vi "430_TCP_compound query test.vi"() -> ()   [LabVIEW 2011]
panel:
  out "refnum out":refnum<file>
  out "file check":errorcluster
  in  "file path (use dialog)":path
  in  "save":bool
  out "status":i32
  in  "Timeout":i32=1000
  out "field":string
  out "Query check":errorcluster
  out "Response":string
  in  "Command":string
  out "Init Response":string
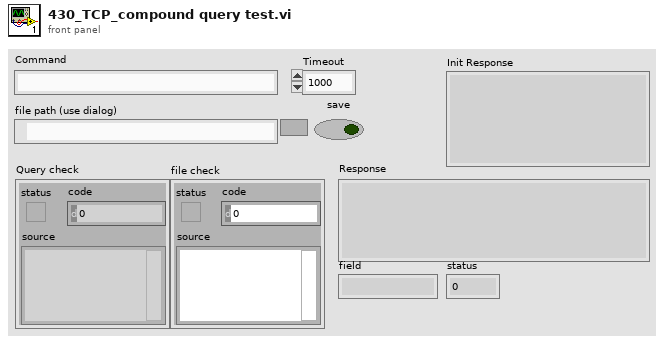
[diagram p1: front panel]
types:
  T1 = enum16{"open", "replace", "create", "open or create", "replace or create", "replace or create with confirmation"}
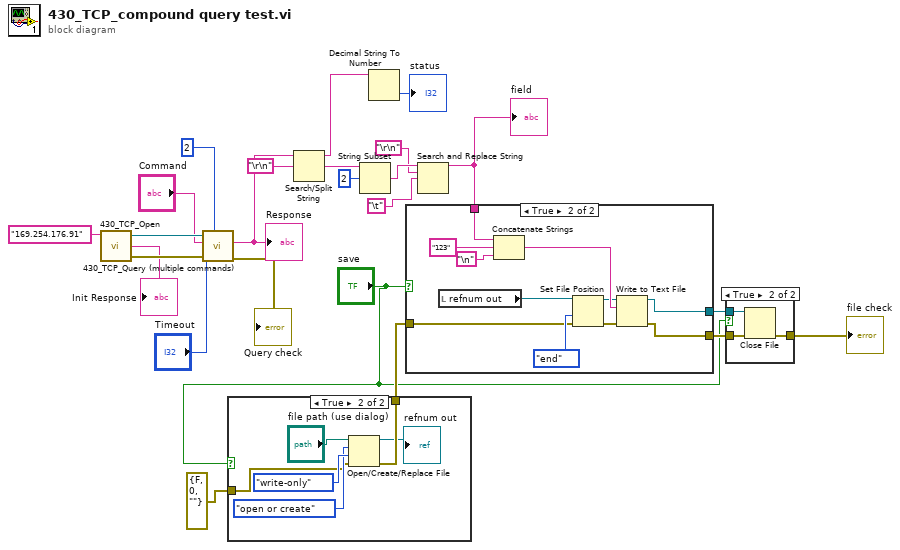
[diagram p0: block diagram]
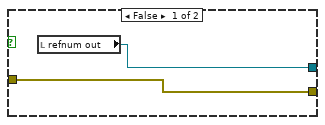
[diagram p4: hidden frame]
diagram:
  n1 = call "430_TCP_Open.vi"("IP Address"="169.254.176.91") -> ("connection ID"=w22:refnum<k5>, "Init Response"=→"Init Response":string, "error out"=w23:errorcluster)  [unwired: 5 in]
  n2 = call "430_TCP_Query (multiple commands).vi"("Number of\nquerys"=2 ("Number of\nquerys"), "error in (no error)"=w23, "Timeout"="Timeout", "Command"="Command", "connection ID"=w22) -> ("error out"=→"Query check":errorcluster, "Response"=w18:string)  [unwired: 2 in, 3 out]
  "Response" <- w18
  n3 = case shown="True" "save" {
    tunnel: [w25 w28] -> w15
    tunnel: errorcluster {"status"=FALSE, "code"=0, "source"=""} ("error out") -> [w25 w26]
    frame False {
    }
    frame True {
      n4 = Open/Create/Replace File(file path (use dialog)="file path (use dialog)", error in=w26, operation (0:open)=T1."open or create", access (0:read/write)=enum16{"read/write", "read-only", "write-only"}."write-only") -> (refnum out=→"refnum out":refnum<file>, error out=w28:errorcluster)  [unwired: 2 in, 1 out]
    }
  }
  n5 = Search/Split String(string=w18, search string/char (-)="\r\n") -> (substring before match=w8:string, match + rest of string=w5:string)  [unwired: 1 in, 1 out]
  n6 = String Subset(string=w5, offset (0)=2) -> (substring=w4:string)  [unwired: 1 in]
  n7 = Decimal String To Number(string=w8) -> (number=→"status":i32)  [unwired: 2 in, 1 out]
  n8 = Search and Replace String(input string=w4, search string="\r\n", replace string="\t") -> (result string=w1:string)  [unwired: 5 in, 3 out]
  "field" <- w1
  n9 = case shown="True" "save" {
    tunnel: [w33 w39] -> w13
    tunnel: w15 -> [w33 w40]
    tunnel: [w32 w38] -> w12
    tunnel: w1 -> [_ w35]
    frame False {
      n10 = local read "refnum out"() -> (w32:refnum<file>)
    }
    frame True {
      n11 = local read "refnum out"() -> (w37:refnum<file>)
      n12 = Concatenate Strings(w35, "123" ("string"), "\n") -> (w44:string)
      n13 = Set File Position(refnum=w37, from (0:start)=enum16{"start", "end", "current"}."end", error in=w40) -> (refnum out=w43:refnum<file>, error out=w41:errorcluster)  [unwired: 1 in]
      n14 = Write to Text File(file (use dialog)=w43, text=w44, error in=w41) -> (refnum out=w38:refnum<file>, error out=w39:errorcluster)  [unwired: 1 in, 1 out]
    }
  }
  n15 = case shown="True" "save" {
    tunnel: [w45 w48] -> w14
    tunnel: w13 -> [w45 w47]
    tunnel: w12 -> [_ w46]
    frame False {
    }
    frame True {
      n16 = Close File(refnum=w46, error in=w47) -> (error out=w48:errorcluster)  [unwired: 1 out]
    }
  }
  "file check" <- w14
